vi "Get File Name.vi"() -> (0 "?":path)   [LabVIEW 2020]
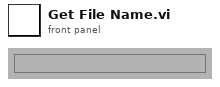
[diagram p1: front panel]
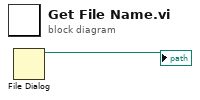
[diagram p0: block diagram]
diagram:
  n1 = File Dialog() -> (3:→"?":path)  [unwired: 7 in, 3 out]
